vi "Approximately equal.vi"(9 "tolerance":dbl=1.0 format="%.2f", 10 "actual":dbl=99.0 format="%.5e", 11 "target":dbl=100.0 format="%.5e") -> (1 "delta":dbl=1.0, 2 "equal?":bool=TRUE)   [LabVIEW 2010]
doc: "Is target and actual equal within tolerance?"
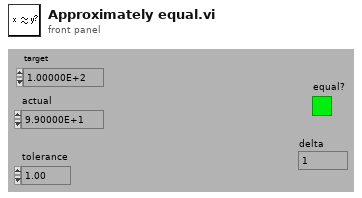
[diagram p1: front panel]
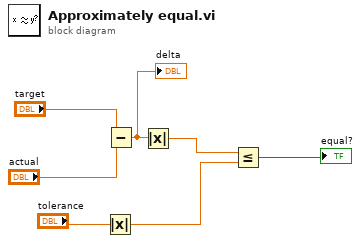
[diagram p0: block diagram]
diagram:
  n1 = Absolute Value(x="tolerance") -> (abs(x)=w2:dbl)
  n2 = Subtract(x="target", y="actual") -> (x-y=w5:dbl)
  "delta" <- w5
  n3 = Absolute Value(x=w5) -> (abs(x)=w7:dbl)
  n4 = Less Or Equal?(x=w7, y=w2) -> (x <= y?=→"equal?":bool)
